vi "FFT Waveform.vi"(8 "error in (no error)":errorcluster, 11 "Waveform in":refnum<class "Waveform.lvclass">) -> (0 "error out":errorcluster, 3 "Waveform out":refnum<class "Waveform.lvclass">)   [LabVIEW 2011, in "Waveform.lvclass"]
uses:
  Waveform.lvclass
  <vilib>/express/express analysis/Spectral/Block/exnSpectralBlock spectral measurements power poly.vi
  <vilib>/express/express analysis/Spectral/Block/exnSpectralBlock spectral measurements power WFM.vi
  <vilib>/express/express analysis/Spectral/XNode/ExpressSpectralMeasurementsBlockNode.xnode
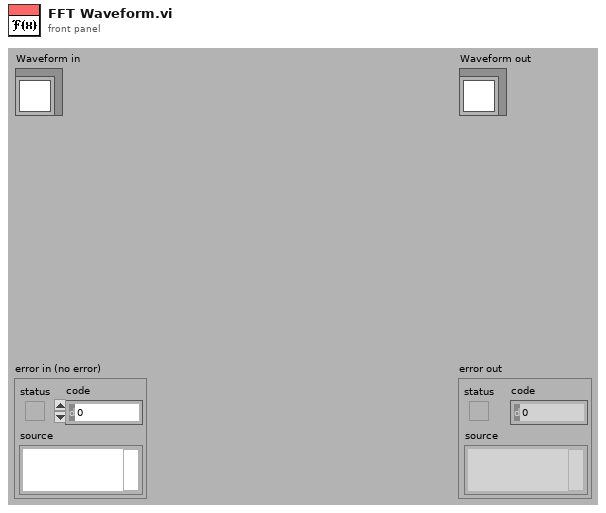
[diagram p1: front panel]
types:
  T1 = cluster{"averaging mode":u16, "weighting mode":u16, "number of averages":u32}
  T2 = cluster{"dB On (F)":bool, "unwrap phase (F)":bool, "convert to degree (F)":bool}
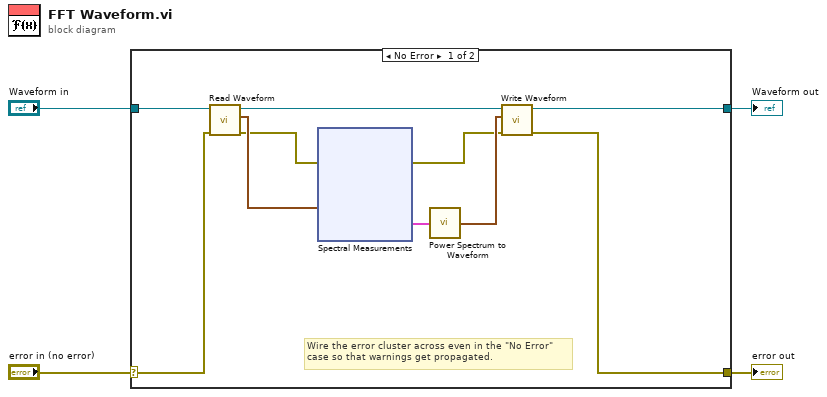
[diagram p0: block diagram]
diagram:
  n1 = case shown="No Error" "error in (no error)" {
    selector: "error in (no error)" -> [w5 w25]
    tunnel: [w6 w25] -> w3
    tunnel: [w9 w24] -> w1
    tunnel: "Waveform in" -> [w14 w24]
    frame No Error {
      # "Wire the error cluster across even in the \"No Error\"\ncase so that warnings get propagated."
      n2 = call-dynamic "Read Waveform.vi"("error in (no error)"=w5, "Waveform in"=w14) -> ("error out"=w12:errorcluster, "Waveform"=w13:waveform(dbl), "Waveform out"=w10:refnum<class "Waveform.lvclass">)  [unwired: 7 in]
      n3 = xnode "Spectral Measurements"("Signals"=w13, "error in (no error)"=w12) -> ("Power Spectrum"=w11:cluster{"f0":dbl, "df":dbl, "magnitude":dbl[]}, "error out"=w7:errorcluster)
      n4 = call "Power Spectrum to Waveform.vi"("Power Spectrum"=w11) -> ("Waveform"=w8:waveform(dbl))
      n5 = call-dynamic "Write Waveform.vi"("error in (no error)"=w7, "Waveform"=w8, "Waveform in"=w10) -> ("error out"=w6:errorcluster, "Waveform out"=w9:refnum<class "Waveform.lvclass">)  [unwired: 7 in]
    }
    frame Error {
    }
  }
  "error out" <- w3
  "Waveform out" <- w1
